vi "Get All Data.vi"(8 "error in (no error)":errorcluster, 11 "List in":refnum<class "List.lvclass">) -> (0 "error out":errorcluster, 2 "data":dbl[](array[numeric]), 3 "List out":refnum<class "List.lvclass">)   [LabVIEW 2021, in "List.lvclass"]
doc: "本VI是为《我和LabVIEW》一书编写的示例。\n关于本书的介绍请参考网页：\nhttp://ruanqizhen.spaces.live.com/blog/cns!5852D4F797C53FB6!4310.entry"
uses:
  List.lvclass
  List.lvclass/List.ctl
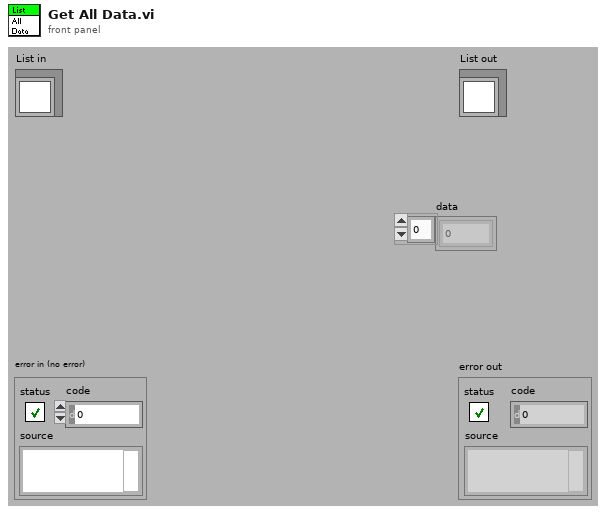
[diagram p1: front panel]
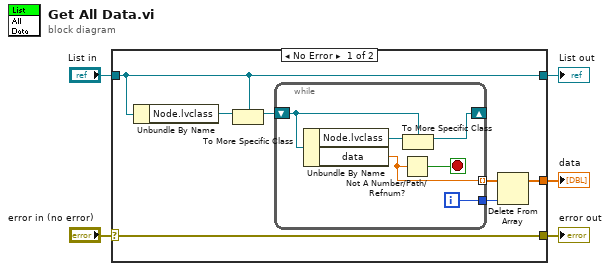
[diagram p0: block diagram]
diagram:
  n1 = case shown="No Error" "error in (no error)" {
    selector: "error in (no error)" -> [w12 w20]
    tunnel: [w12 w20] -> w4
    tunnel: [w10 w19] -> w2
    tunnel: "List in" -> [w10 w19]
    tunnel: [w6 _] -> w1
    frame No Error {
      n2 = Unbundle By Name(w10) -> ("Node.lvclass"=w11:refnum<class "Node.lvclass">)
      n3 = To More Specific Class(target class=w10, reference=w11) -> (specific class reference=w9:refnum<class "List.lvclass">)  [unwired: 1 in, 1 out]
      n4 = while {
        shift-right: [w16] -> _
        shift-left: w9 -> [w18]
        tunnel: [w14] -> w7 mode=indexing
        tunnel: [w13] -> w8
        i -> [w13]
        stop <- w15 stop-if-true
        n5 = Unbundle By Name(w18) -> ("Node.lvclass"=w17:refnum<class "Node.lvclass">, "data"=w14:dbl)
        n6 = Not A Number/Path/Refnum?(number/path/refnum=w14) -> (NaN/Path/Refnum?=w15:bool)
        n7 = To More Specific Class(target class=w18, reference=w17) -> (specific class reference=w16:refnum<class "List.lvclass">)  [unwired: 1 in, 1 out]
      }
      n8 = Delete From Array(array=w7, index=w8) -> (array with subset deleted=w6:dbl[])  [unwired: 1 in, 1 out]
    }
    frame Error {
    }
  }
  "error out" <- w4
  "List out" <- w2
  "data" <- w1
